vi "FFT on data.vi"(5 "dt":dbl, 6 "Data":dbl[](array[numeric])) -> (0 "XY Graph":cluster{dbl[], "magnitude":dbl[]}(graph), 1 "FFT {X}":cdb[](array[numeric]), 2 "abs FFT":dbl[](graph), 3 "output":dbl[][](array[numeric]), 4 "frequency (Hz)":dbl[](array[numeric]))   [LabVIEW 2009]
uses:
  <vilib>/measure/maspectr.llb/FFT Power Spectrum for N Chan.vi
  <vilib>/Analysis/2dsp.llb/Real FFT.vi
  <vilib>/measure/NI_MAPro.lvlib
  <vilib>/Analysis/NI_AALPro.lvlib
panel:
  out "df":dbl
  out "Waveform Graph":dbl[](graph)
  out "Sensor 2 ax":cluster{"f0":dbl, "df":dbl, "magnitude":dbl[]}[](graph)
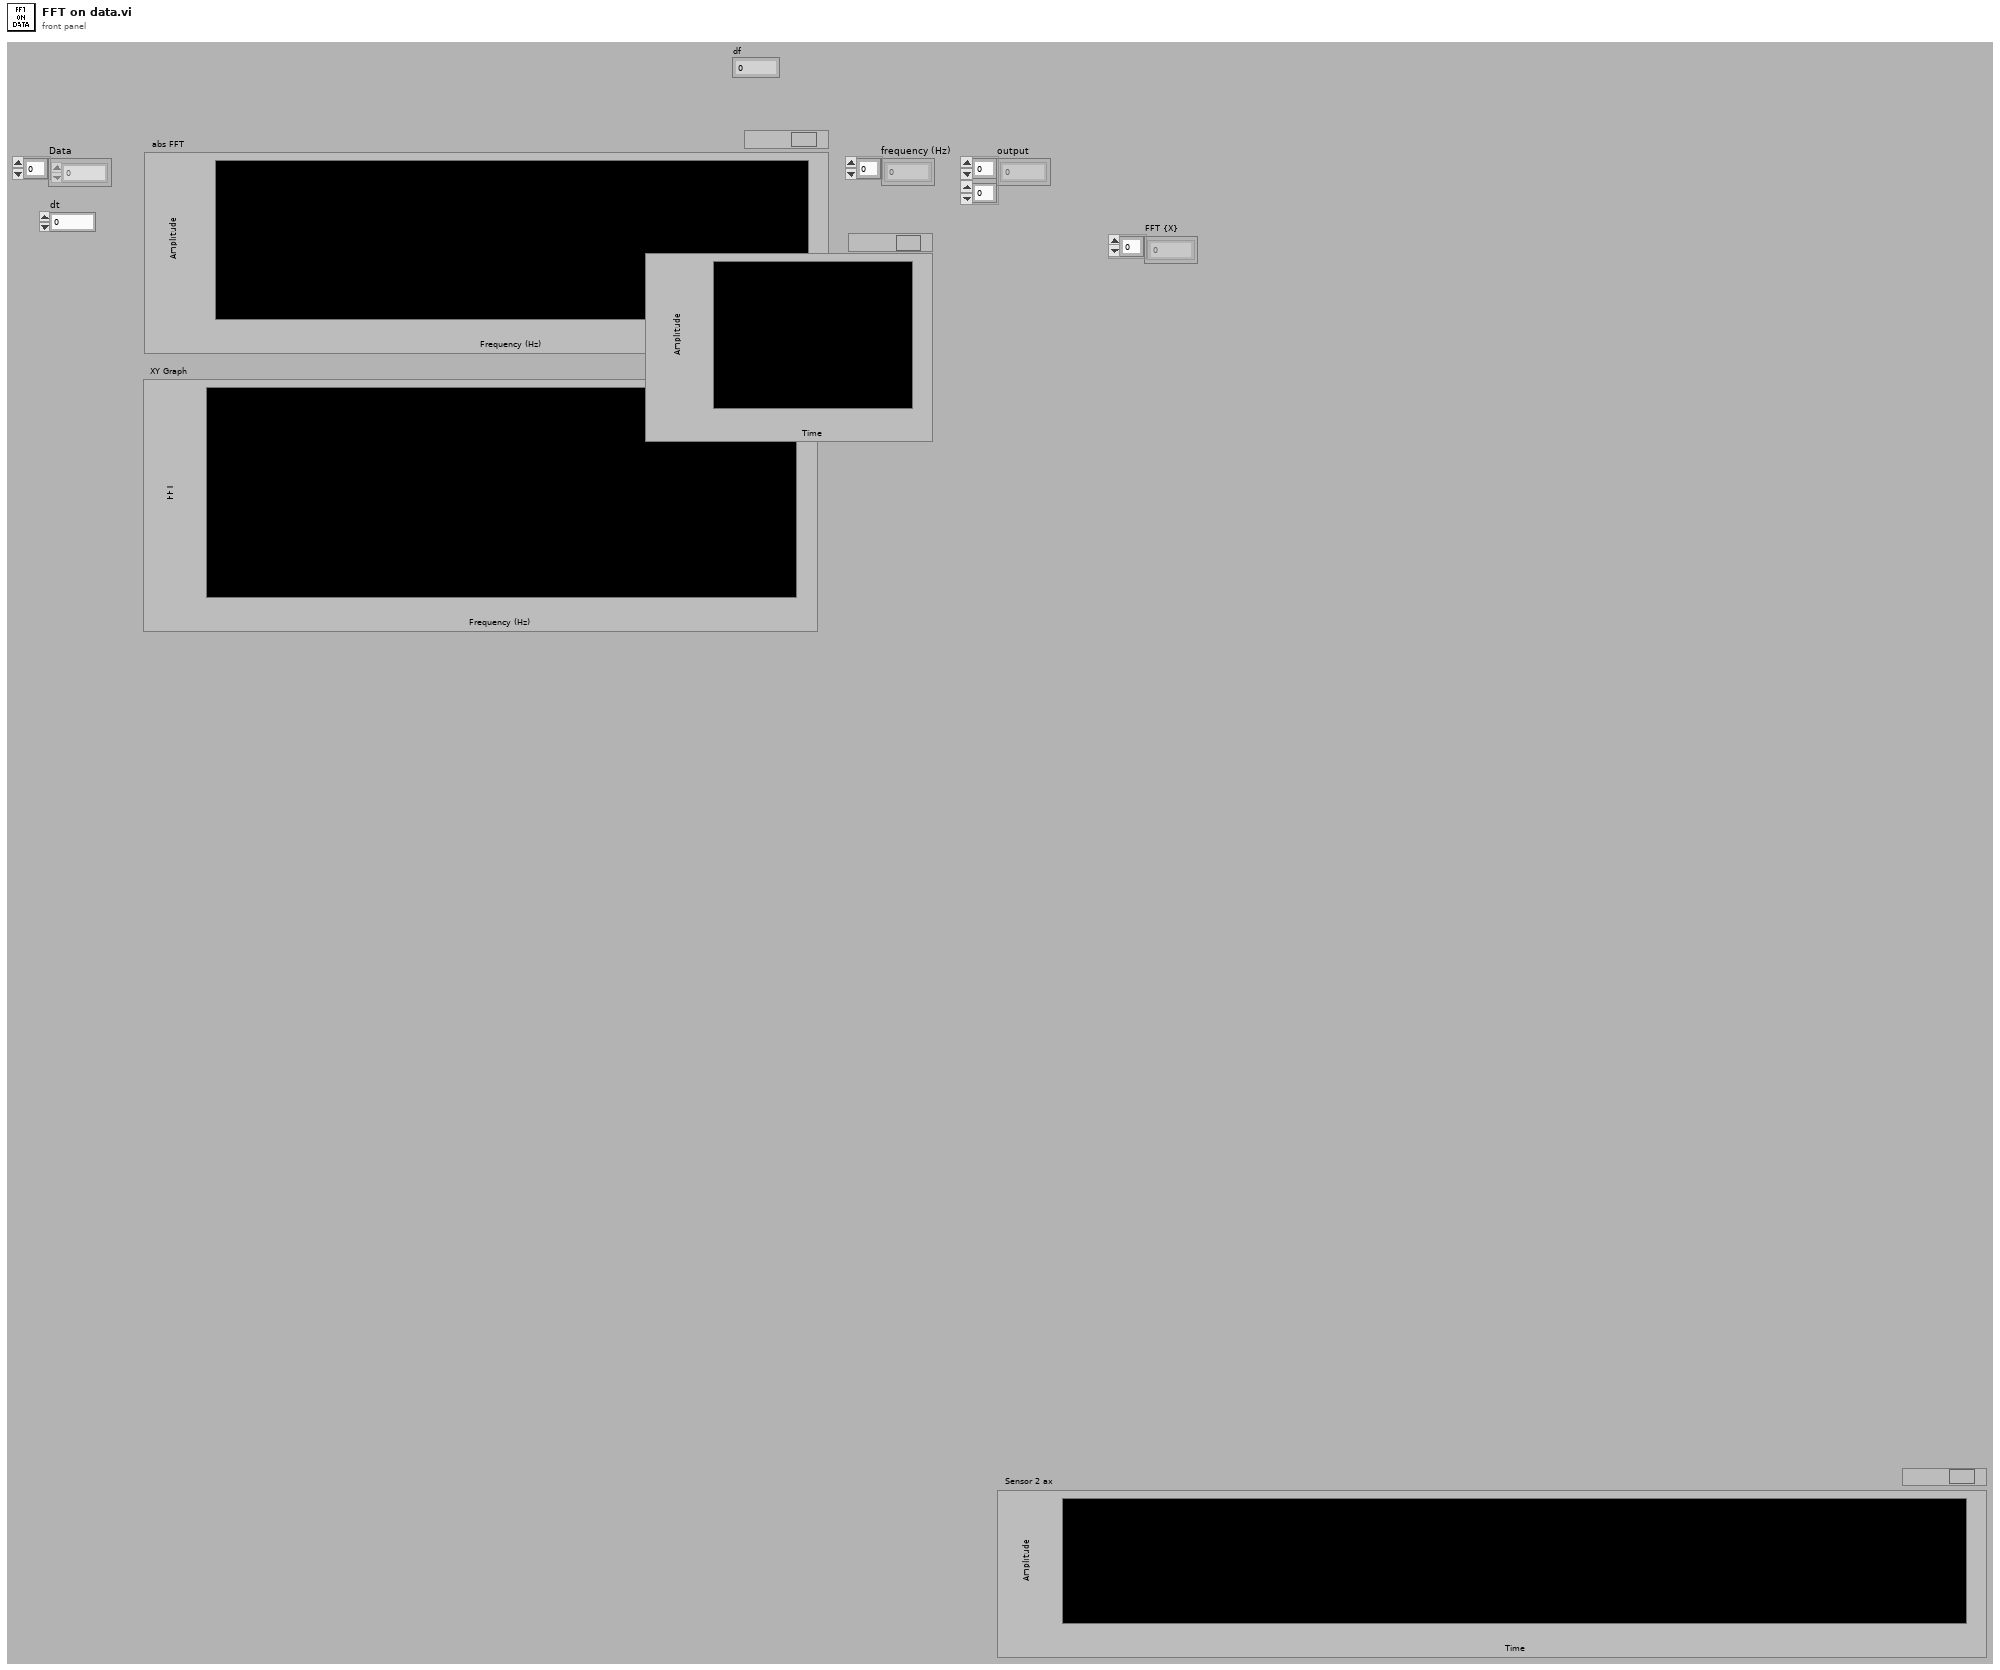
[diagram p1: front panel]
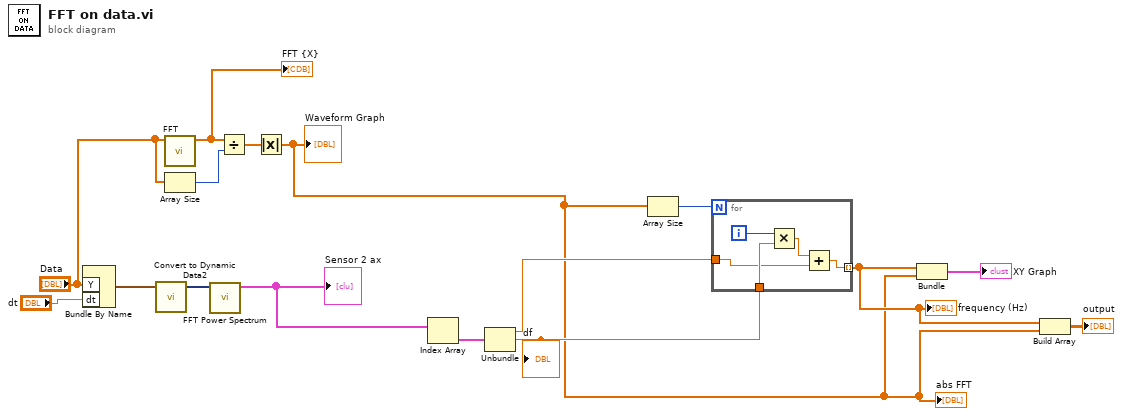
[diagram p0: block diagram]
diagram:
  n1 = Bundle By Name("Y"="Data", "dt"="dt") -> (w7:waveform(dbl))  [unwired: 1 in]
  n2 = call "Convert to Dynamic Data2"("Waveform"=w7) -> ("Dynamic Data Type"=w16:dynamicdata)  [unwired: 3 in]
  n3 = call-poly <vilib>:"FFT.vi"("X"="Data") -> ("FFT {X}"=w4:cdb[])  [unwired: 9 in, 1 out]
  "FFT {X}" <- w4
  n4 = Array Size(array="Data") -> (size(s)=w5:i32)
  n5 = call-poly <vilib>:"FFT Power Spectrum.vi"("time signals"=w16) -> ("power spectra"=w14:cluster{"f0":dbl, "df":dbl, "magnitude":dbl[]}[])  [unwired: 7 in, 3 out]
  "Sensor 2 ax" <- w14
  n6 = Divide(x=w4, y=w5) -> (x/y=w3:cdb[])
  n7 = Absolute Value(x=w3) -> (abs(x)=w1:dbl[])
  "abs FFT" <- w1
  "Waveform Graph" <- w1
  n8 = Index Array(array=w14) -> (element=w15:cluster{"f0":dbl, "df":dbl, "magnitude":dbl[]})  [unwired: 1 in]
  n9 = Unbundle(w15) -> ("f0"=w13:dbl, "df"=w12:dbl)  [unwired: 1 out]
  "df" <- w12
  n10 = Array Size(array=w1) -> (size(s)=w2:i32)
  n11 = for {
    N: w2 -> [_]
    tunnel: w13 -> [w18]
    tunnel: w12 -> [w21]
    tunnel: [w19] -> w9 mode=indexing
    i -> [w17]
    n12 = Multiply(x=w17, y=w21) -> (x*y=w20:dbl)
    n13 = Add(x=w20, y=w18) -> (x+y=w19:dbl)
  }
  "frequency (Hz)" <- w9
  n14 = Bundle(w9, w1) -> (→"XY Graph":cluster{dbl[], dbl[]})  [unwired: 1 in]
  n15 = Build Array(w9, w1) -> (→"output":dbl[][])
